vi "FPGA_AIWriteAverageBits.vi"(8 "error in (no error)":errorcluster, 9 "AverageBit":u8, 10 "Channel":T1=enum."AI 1", 11 "AI Reference in":T2) -> (0 "error out":errorcluster, 3 "AI Reference out":T2)   [LabVIEW 2017]
uses:
  <vilib>/Rock Robotics/SystemInterfaces/AI/FPGA_AIDevRef.ctl
  <vilib>/Rock Robotics/SystemInterfaces/AI/FPGA_AIChannel.ctl
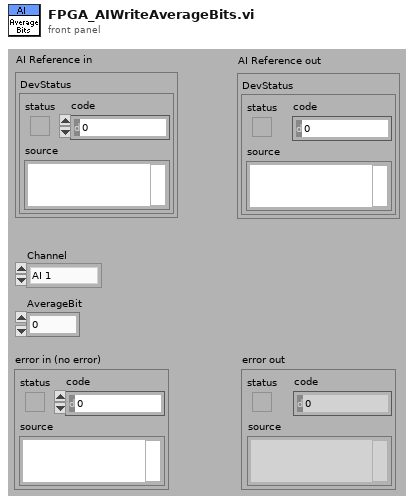
[diagram p1: front panel]
types:
  T1 = typedef "FPGA_AIChannel.ctl" = enum8{"AI 0", "AI 1", "AI 2", "AI 3", "AI MXP 0", "AI MXP 1", "AI MXP 2", "AI MXP 3", "Invalid"}
  T2 = typedef "FPGA_AIDevRef.ctl" = cluster{"DevStatus":errorcluster}
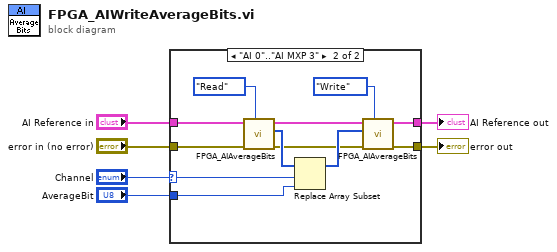
[diagram p0: block diagram]
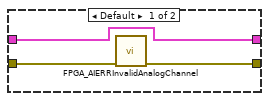
[diagram p2: hidden frame]
diagram:
  n1 = case shown="\"AI 0\"..\"AI MXP 3\"" "Channel" {
    selector: "Channel" -> [_ w18]
    tunnel: "AI Reference in" -> [w7 w21]
    tunnel: "error in (no error)" -> [w9 w20]
    tunnel: "AverageBit" -> [_ w17]
    tunnel: [w7 w13] -> w2
    tunnel: [w8 w12] -> w1
    frame Default {
      n2 = call <vilib>:"FPGA_AIERRInvalidAnalogChannel.vi"("error in (no error)"=w9) -> ("error out"=w8:errorcluster)  [unwired: 10 in]
    }
    frame "AI 0".."AI MXP 3" {
      n3 = call <vilib>:"FPGA_AIAverageBits.vi"("Task"=enum16{"Read", "Write"}."Read", "error in (no error)"=w20, "AI Reference in"=w21) -> ("error out"=w14:errorcluster, "AverageBits out"=w19:u8[], "AI Reference out"=w15:T2)  [unwired: 2 in, 4 out]
      n4 = Replace Array Subset(array=w19, new element=w17, index=w18) -> (w16:u8[])
      n5 = call <vilib>:"FPGA_AIAverageBits.vi"("Task"=enum16{"Read", "Write"}."Write", "error in (no error)"=w14, "AverageBits in"=w16, "AI Reference in"=w15) -> ("error out"=w12:errorcluster, "AI Reference out"=w13:T2)  [unwired: 6 out]
    }
  }
  "AI Reference out" <- w2
  "error out" <- w1
